vi "Error Cleanup.vi"(8 "error in (no error)":errorcluster, 11 "Protocol Parent in":refnum<class "Protocol Parent.lvclass">) -> (0 "error out":errorcluster, 3 "Protocol Parent out":refnum<class "Protocol Parent.lvclass">)   [LabVIEW 2023, in "Protocols.lvlib" / "Protocol Parent.lvclass"]
uses:
  Protocol Parent.lvclass
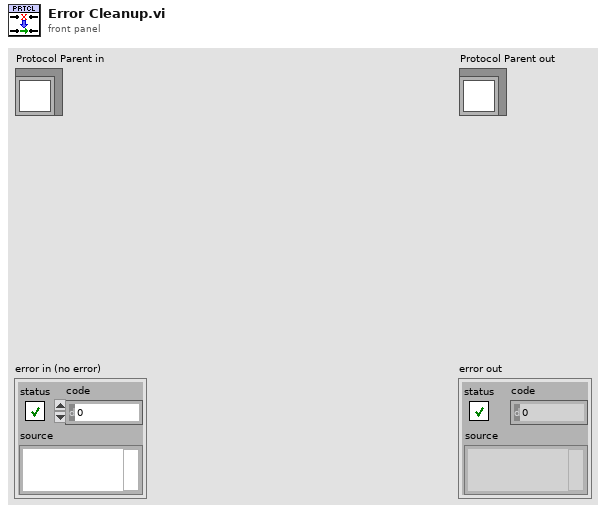
[diagram p1: front panel]
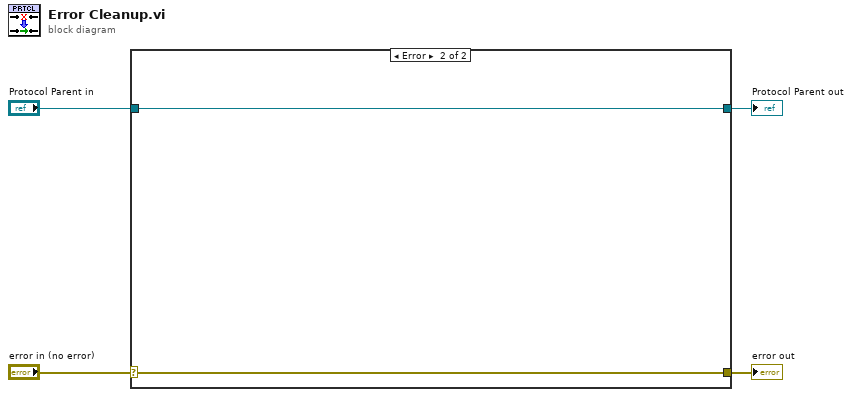
[diagram p0: block diagram]
diagram:
  n1 = case shown="Error" "error in (no error)" {
    selector: "error in (no error)" -> [w5 w8]
    tunnel: [w5 w8] -> w3
    tunnel: [w6 w7] -> w1
    tunnel: "Protocol Parent in" -> [w6 w7]
    frame No Error {
      # "Wire the error cluster across even in the \"No Error\"\ncase so that warnings get propagated."
    }
    frame Error {
    }
  }
  "error out" <- w3
  "Protocol Parent out" <- w1
